vi "Get Word Ref.vi"(8 "error in (no error)":errorcluster, 11 "MS-Word in":refnum<class "MS-Word.lvclass">) -> (0 "error out":errorcluster, 2 "Word Ref":refnum<k24>, 3 "MS-Word out":refnum<class "MS-Word.lvclass">)   [LabVIEW 2017, in "LabVIEW NPOI.lvlib" / "MS-Word.lvclass"]
uses:
  MS-Word.lvclass
  C:/Users/Neo/Desktop/Dev_Tools_BR/LabVIEW_NPOI/src/lib/NPOI 2.1.1/NPOI.OOXML.dll
  lib/NPOI 2.1.1/NPOI.OOXML.dll
  MS-Word.lvclass/MS-Word.ctl
  xwpfDocument/xwpfDocument.lvclass/xwpfDocument.ctl
  xwpfDocument/Get Document.Ref.vi
  xwpfDocument/xwpfDocument.lvclass
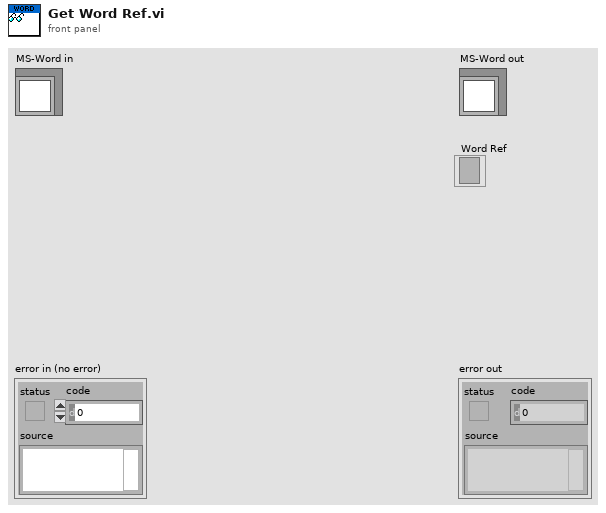
[diagram p1: front panel]
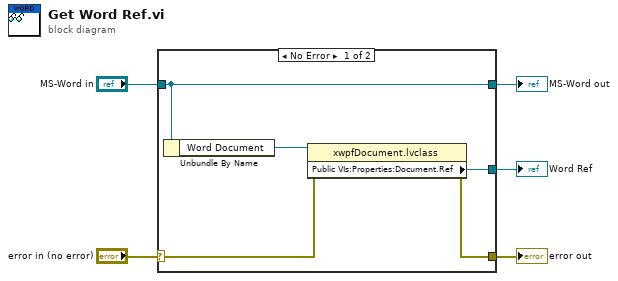
[diagram p0: block diagram]
diagram:
  n1 = case shown="No Error" "error in (no error)" {
    selector: "error in (no error)" -> [w7 w11]
    tunnel: [w6 w11] -> w4
    tunnel: [w10 w12] -> w2
    tunnel: "MS-Word in" -> [w10 w12]
    tunnel: [w8 _] -> w1
    frame No Error {
      n2 = Unbundle By Name(w10) -> ("Word Document"=w9:refnum<class "xwpfDocument.lvclass">)
      n3 = property class="xwpfDocument.lvclass"(reference=w9, error in=w7) -> (error out=w6:errorcluster, "Public VIs:Properties:Document.Ref"=w8:refnum<k24>)  [unwired: 1 out]
    }
    frame Error {
    }
  }
  "error out" <- w4
  "MS-Word out" <- w2
  "Word Ref" <- w1
